vi "BL_GetChannelsPlugged .vi"(8 "error in (no error)":errorcluster, 11 "Potentiostat Galvanostat in":refnum<class "Potentiostat Galvanostat.lvclass">) -> (0 "error out":errorcluster, 2 "Plugged Channels":u8[](array[numeric]), 3 "Potentiostat Galvanostat out":refnum<class "Potentiostat Galvanostat.lvclass">)   [LabVIEW 2018, in "Potentiostat Galvanostat.lvclass"]
doc: "This function tests the communication speed between the library and the selected channel. \nNOTE: This function is for advanced user only."
uses:
  Potentiostat Galvanostat.lvclass
  Potentiostat Galvanostat.lvclass/Potentiostat Galvanostat.ctl
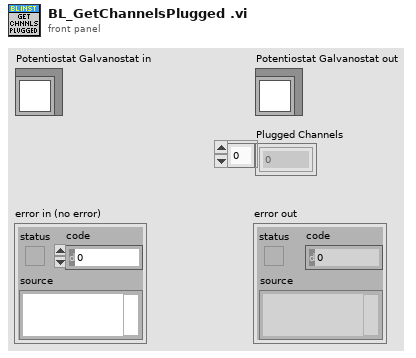
[diagram p1: front panel]
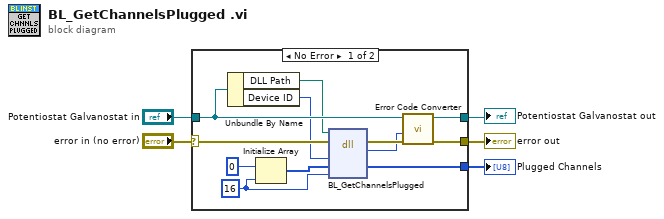
[diagram p0: block diagram]
diagram:
  n1 = case shown="No Error" "error in (no error)" {
    selector: "error in (no error)" -> [w11 w19]
    tunnel: [w17 w19] -> w4
    tunnel: [w16 w18] -> w2
    tunnel: "Potentiostat Galvanostat in" -> [w15 w18]
    tunnel: [w6 _] -> w1
    frame No Error {
      w12 = 16 ("dimension size")
      n2 = Unbundle By Name(w15) -> ("DLL Path"=w9:path, "Device ID"=w10:i32)
      n3 = Initialize Array(u8 0 ("element"), w12) -> (w14:u8[])
      n4 = dll-call lib="C:/Program Files (x86)/National Instruments/LabVIEW 2018/user.lib/EClib/EClib.*" fn="BL_GetChannelsPlugged"(path in=w9, error in=w11, "Device ID"=w10, "Plugged Channels"=w14, "Size"=w12) -> (error out=w8:errorcluster, "Error Code"=w7:i32, "Plugged Channels"=w6:u8[])  [unwired: 3 in, 1 out]
      n5 = call-dynamic "Error Code Converter.vi"("error in (no error)"=w8, "Error Code"=w7, "Potentiostat Galvanostat in"=w15) -> ("error out"=w17:errorcluster, "Potentiostat Galvanostat out"=w16:refnum<class "Potentiostat Galvanostat.lvclass">)  [unwired: 7 in]
    }
    frame Error {
    }
  }
  "error out" <- w4
  "Potentiostat Galvanostat out" <- w2
  "Plugged Channels" <- w1
